vi "pigeon_ver4_1.vi"() -> ()   [LabVIEW 2017]
uses:
  <vilib>/eio/EIONode/EIONode.xnode
  <vilib>/Platform/TimedLoop/XDataNode/XDataNode.xnode
  <vilib>/Platform/TimedLoop/XDataNode/nitl_modes.ctl
  <vilib>/Platform/TimedLoop/XDataNode/XDNodeRunTimeDep.lvlib
  <vilib>/Platform/TimedLoop/XDataNode/wakeup.ctl
  <vilib>/Platform/TimedLoop/XDataNode/timing_clust.ctl
  <vilib>/rvi/DataTransferAndStorage/Container/XNode/niFpgaContainer.xnode
  <vilib>/rvi/eio/common/nirviEmuTemplateMethod_errors.vi
  <vilib>/rvi/Memory/Memory_Emulation/nirvimemoryFastEmulation.vi
  <vilib>/rvi/Memory/Memory_Emulation/nirvimemoryEmulation.vi
  <vilib>/rvi/interface/RandomDataEmulation/nirviRandomDataFpgaReadWriteTemplate.vi
panel:
  out "Numeric":i16
  in  "analog ramp on":bool
  in  "AO5":i16
  out "AI2":i16
  in  "Tab Control":enum32{"pigeon"}(tab)
  out "trigger AI1":bool
  in  "Tab Control 2":T1(tab)
  in  "square wave  on?":bool
  in  "square wave period":i32
  in  "IGBTswitch":bool caption="IGBT Switch circular"
  in  "Manual Override":bool
  in  "circular coil current":i16(slide) scale=0.0..32768.0
  in  "analog ramp period":i16
  in  "AO4":bool
  in  "analog wave shape":i16(ring) items=["Triangle", "Sawtooth", "Sin", ""]
  out "FIFO size":i16
  in  "AO0":i16
  in  "AO1":i16
  in  "AO2":i16
  in  "Run program":bool
  in  "halt processor":bool
  out "control flags":i8 format="%b"
  in  "host operation":i16
  in  "address":u16
  in  "data1":u16
  in  "data2":i32
  in  "repeat program":i32
  out "IP address":i16
  out "PMT1":i16=-4740
  out "ReA":i32
  out "RegB":i16
  out "RegC":i16
  out "exttrigger":bool=TRUE
  out "AI1":i16=161
  out "RegD":i16
  in  "AO4":i16
  in  "AO3":i16
  out "Connector0/AI0":i16
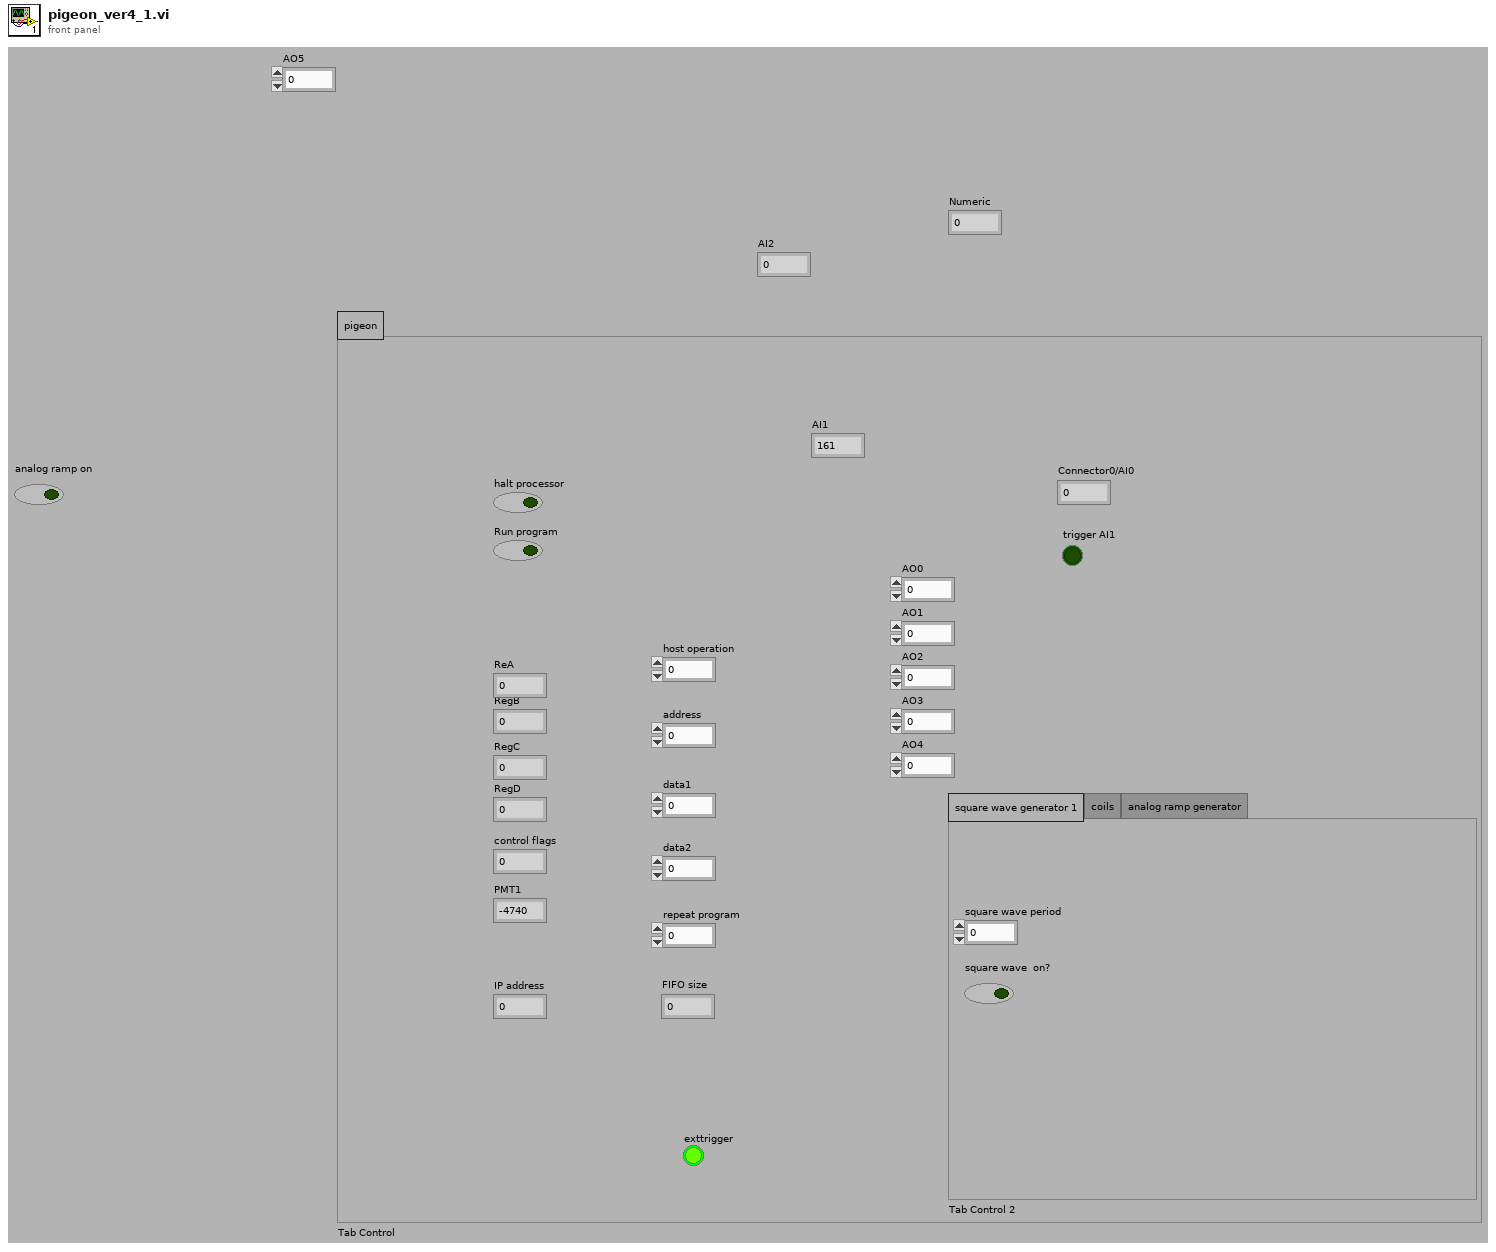
[diagram p1: front panel]
types:
  T1 = enum32{"square wave generator 1", "coils", "analog ramp generator"}
  T2 = typedef "XDNodeRunTimeDep.lvlib/timing_clust.ctl" = cluster{"Expected End [f-1]":u64, "Actual End [f-1]":u64, "Finished Late? [f-1]":bool, "Expected End [i-1]":u64, "Actual End [i-1]":u64, "Finished Late? [i-1]":bool, "Expected Start [i]":u64, "Actual Start [i]":u64, "Expected Start [f]":u64, "Actual Start [f]":u64, "Source Name":string, "Structure Name":string, "Period":i64, "Deadline":i64, "Offset":i64, "Start":i64, "Priority":i32, "Timeout":i32, "Mode":T3, "Wakeup Reason":T4, "Error":errorcluster, "Source Type":string, "Secondary Source Type":string, "Global End Time":u64, "Global Start Time":u64, "Frame Duration":u64, "Iteration Duration":u64, "Assigned CPU":i32, "I/O Scan Engine Mode":u32}
  T3 = typedef "XDNodeRunTimeDep.lvlib/nitl_modes.ctl" = enum32{"No Change", "Process missed periods, maintain original phase", "Discard missed periods, maintain original phase", "Process missed periods, ignore original phase", "Discard missed periods, ignore original phase"}
  T4 = typedef "XDNodeRunTimeDep.lvlib/wakeup.ctl" = enum32{"Normal", "Aborted", "Asynchronous wakeup", "Timing source error", "Timed loop error", "Timeout"}
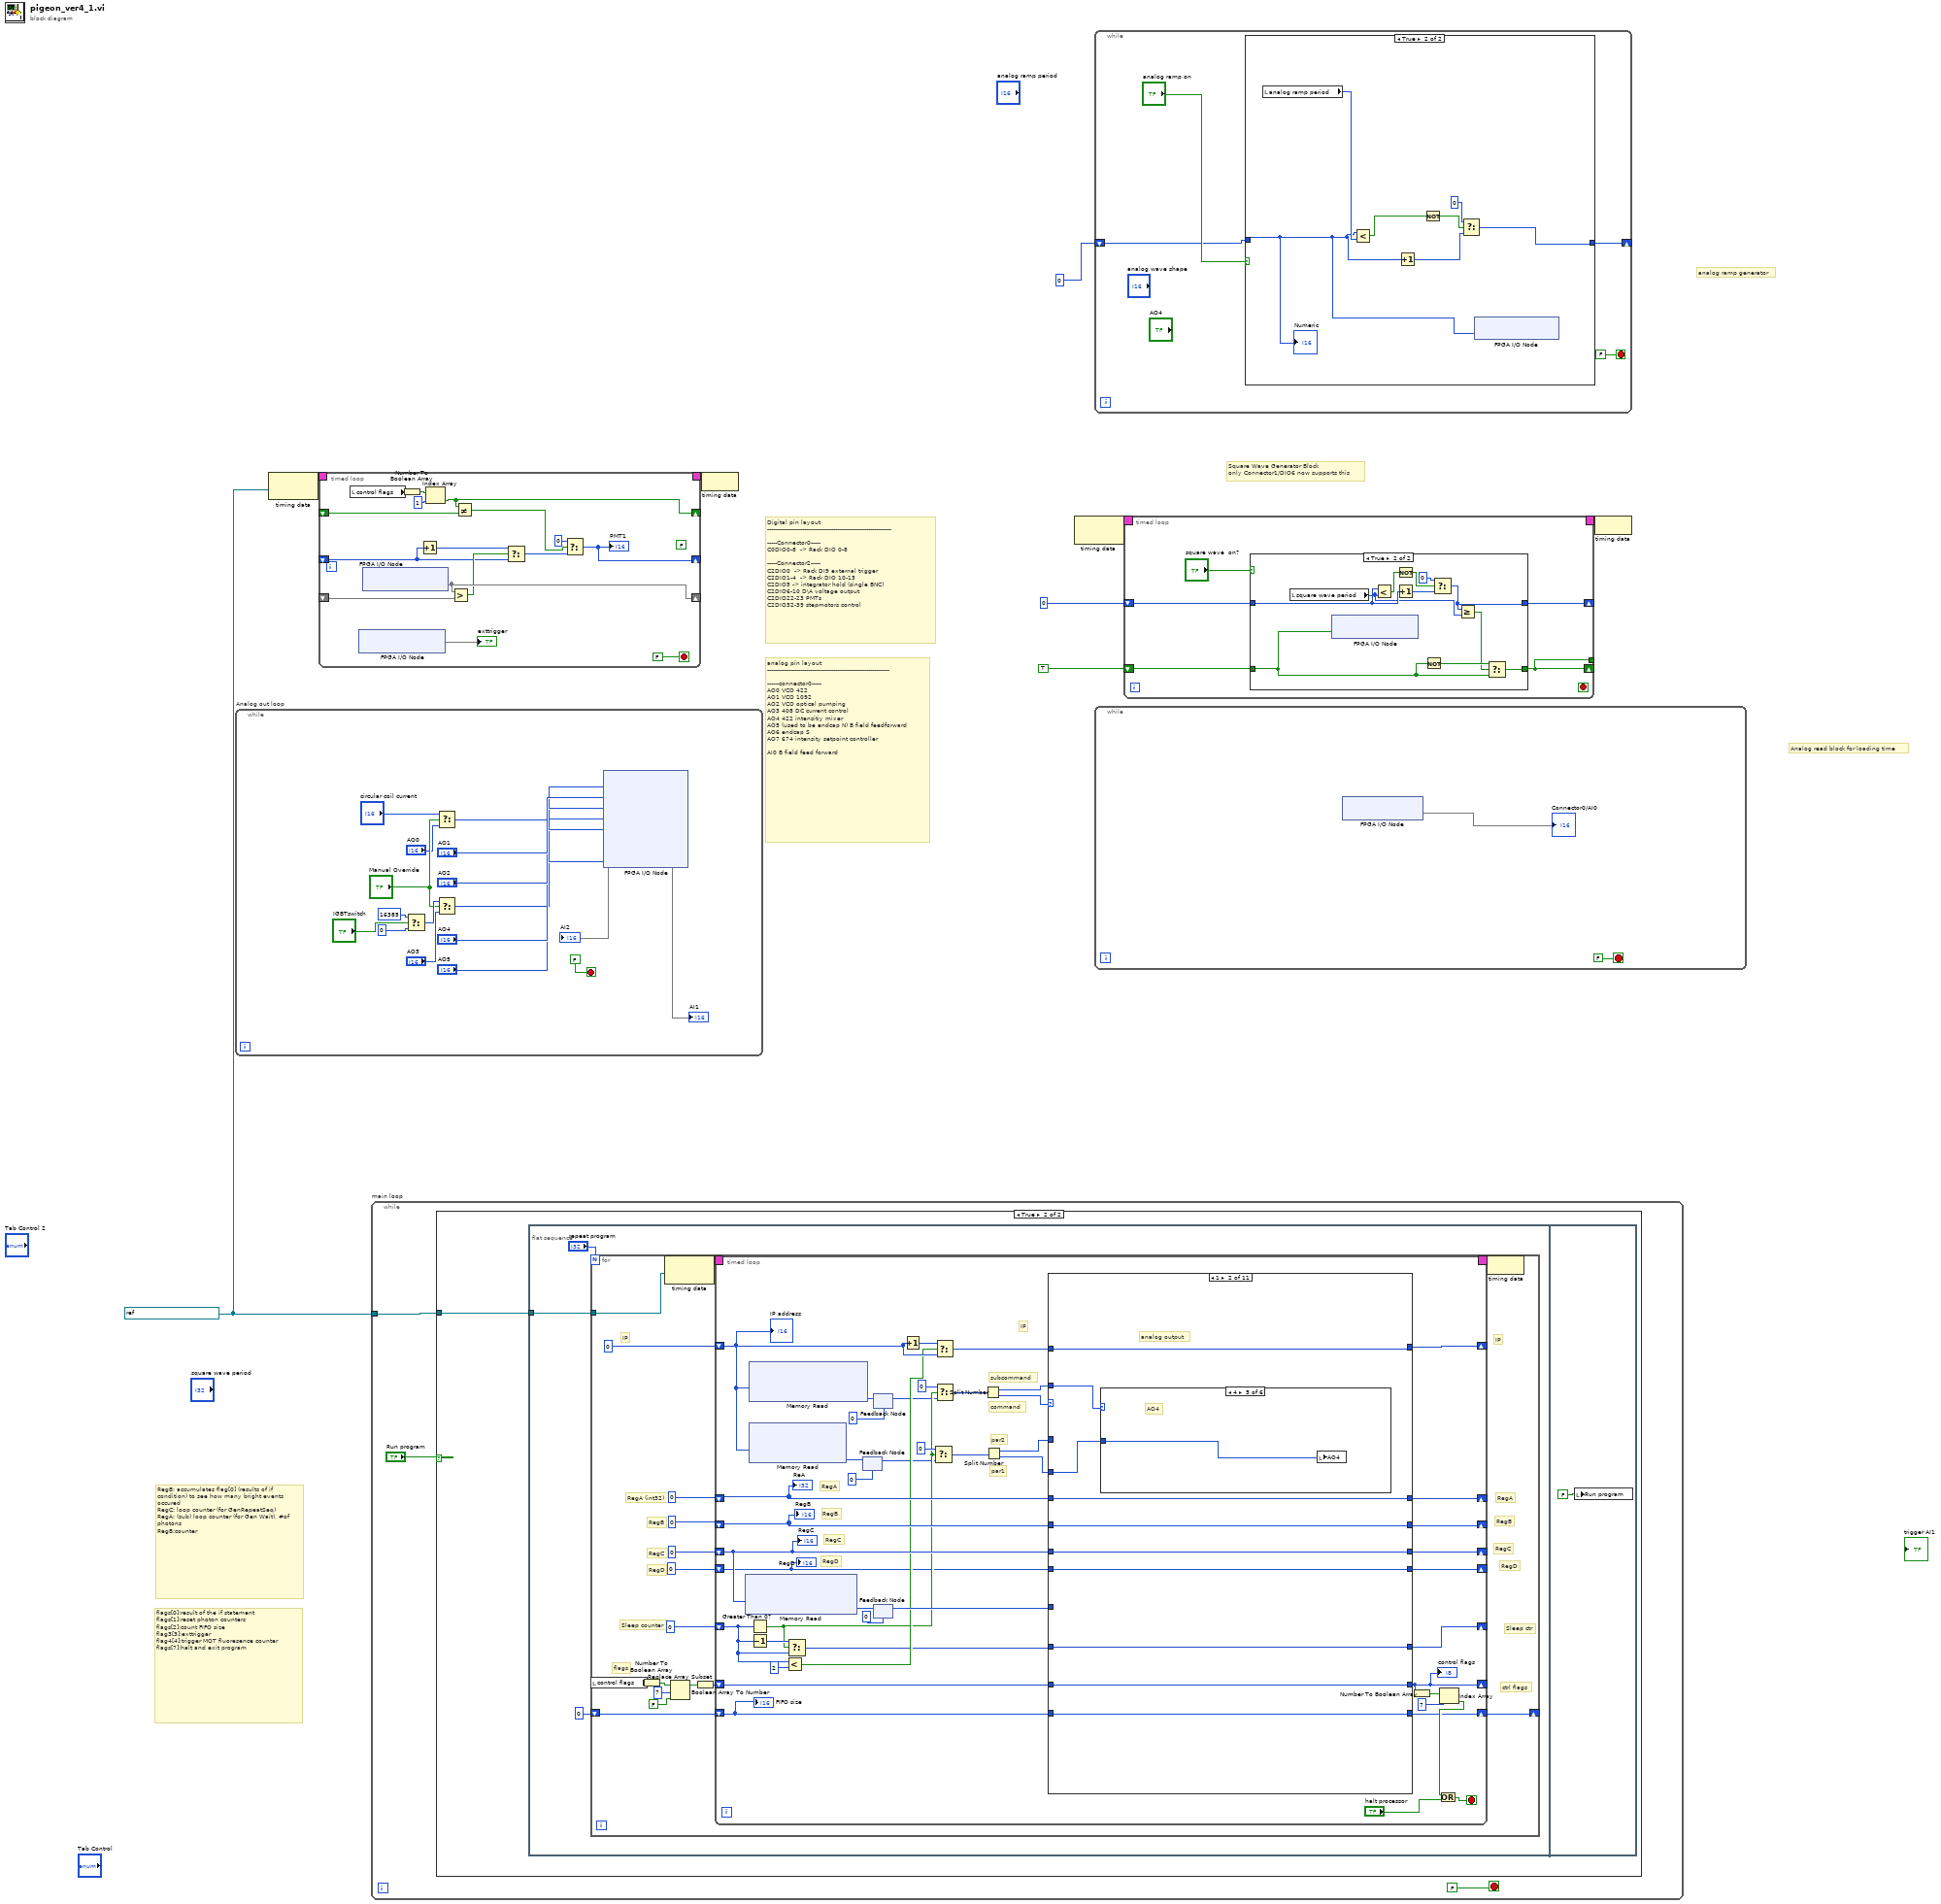
[diagram p0: block diagram]
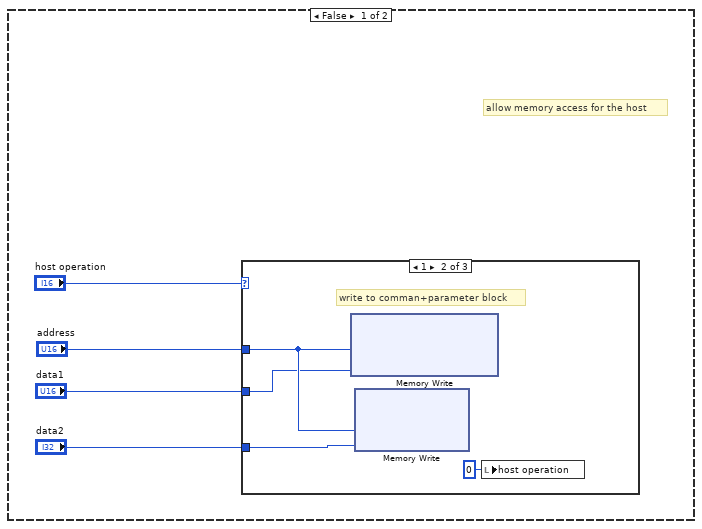
[diagram p4: hidden frame]
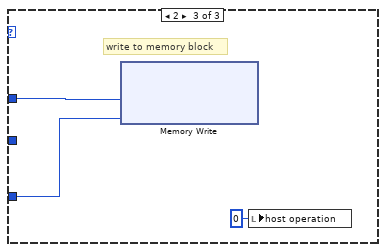
[diagram p6: hidden frame]
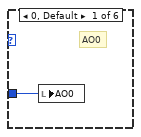
[diagram p8: hidden frame]
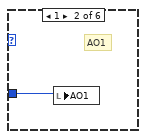
[diagram p9: hidden frame]
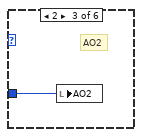
[diagram p10: hidden frame]
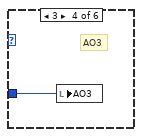
[diagram p11: hidden frame]
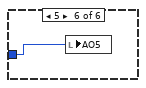
[diagram p12: hidden frame]
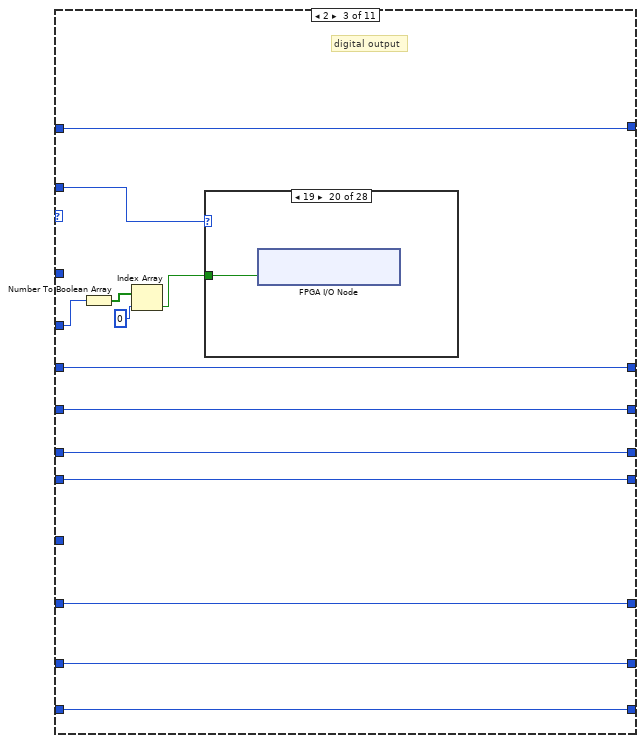
[diagram p13: hidden frame]
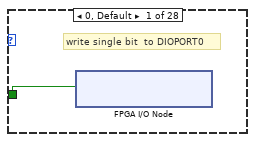
[diagram p14: hidden frame]
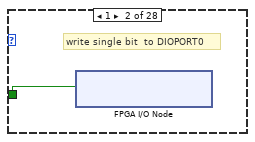
[diagram p15: hidden frame]
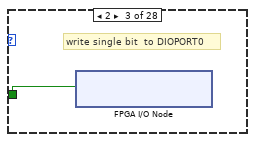
[diagram p16: hidden frame]
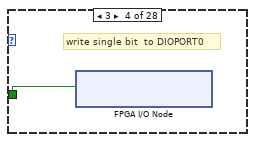
[diagram p17: hidden frame]
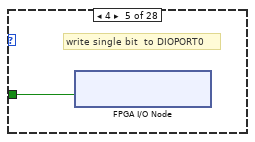
[diagram p18: hidden frame]
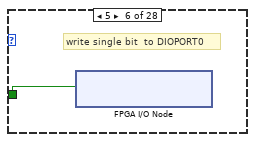
[diagram p19: hidden frame]
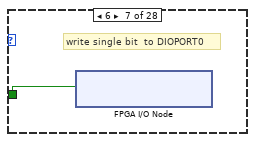
[diagram p20: hidden frame]
diagram:
  w6 = refnum<k21> "40 MHz Onboard Clock" ("FPGA Clock")
  # "analog ramp generator"
  # "Analog read block for loading time"
  # "Square Wave Generator Block\nonly Connector1/DIO6 now supports this"
  # "RegB: accumulates flag[0] (results of if condition) to see how many bright events occured\nRegC: loop counter (for GenRepeatSeq)\nRegA: (sub) loop counter (for Gen Wait), #of     photons \nRegB:counter"
  # "flags[0]:result of the if statement\nflags[1]:reset photon counters\nflags[2]:count FIFO size\nflag3[3]:exttrigger\nflag4[4]:trigger MOT fluoresence counter\nflags[7]:halt and exit program"
  # "Digital pin layout\n----------------------------------------------------------------\n\n-----Connector0-----\nC0DIO0-8  -> Rack DIO 0-8\n\n-----Connector2-----\nC2DIO0  -> Rack DI9 external trigger \nC2DIO1-4  -> Rack DIO 10-13\nC2DIO5 -> integrator hold (single BNC)\nC2DIO6-10 D\\A voltage output\nC2DIO22-23 PMTs\nC2DIO32-39 stepmotors control"
  # "analog pin layout\n---------------------------------------------------------------\n\n------connector0-----\nAO0 VCO 422\nAO1 VCO 1092\nAO2 VCO optical pumping\nAO3 408 DC current control\nAO4 422 intensitiy mixer\nAO5 (used to be endcap N) B field feedforward\nAO6 endcap S\nAO7 674 intensity setpoint controller\n\nAI0 B field feed forward"
  n1 = while "Analog out loop" {
    stop <- FALSE stop-if-true
    n2 = Select(t=i16 16385, s="IGBTswitch", f=i16 0) -> (s? t:f=w15:i16)
    n3 = Select(t="circular coil current", s="Manual Override", f="AO0") -> (s? t:f=w9:i16)
    n4 = Select(t=w15, s="Manual Override", f="AO3") -> (s? t:f=w14:i16)
    n5 = xnode "FPGA I/O Node"("Connector0/AO0"=w9, "Connector0/AO1"="AO1", "Connector0/AO2"="AO2", "Connector0/AO3"=w14, "Connector0/AO4"="AO4", "Connector0/AO5"="AO5") -> ("Connector0/AI1"=→"AI1", "Connector0/AI2"=→"AI2")  [unwired: 8 in, 8 out]
  }
  n6 = node-c288(w6) -> (w8:T2)
  n7 = timed-loop {
    timing: w8 -> [_]
    timing-out: [_] -> w7
    shift-right: [w39] -> _
    shift-left: _ -> [w28]
    shift-right: [w32] -> _
    shift-left: _ -> [w41]
    shift-right: [w34] -> _
    shift-left: _ -> [w35]
    stop <- FALSE stop-if-true
    (unwired) FALSE
    n8 = local read "control flags"() -> (w36:i8)
    n9 = xnode "FPGA I/O Node"() -> ("Connector2/DIO0"=→"exttrigger")  [unwired: 1 in, 1 out]
    n10 = xnode "FPGA I/O Node"() -> ("Connector0/DIO0"=w32)  [unwired: 1 in, 1 out]
    n11 = Number To Boolean Array(number=w36) -> (Boolean array=w37:bool[])
    n12 = Increment(x=w28) -> (x+1=w29:u16)
    n13 = Index Array(array=w37, index=1) -> (element=w34:bool)
    n14 = Greater?(x=w32, y=w41) -> (0:w31:bool)
    n15 = Not Equal?(x=w34, y=w35) -> (x != y?=w26:bool)
    n16 = Select(t=w29, s=w31, f=w28) -> (s? t:f=w40:u16)
    n17 = Select(t=u16 0, s=w26, f=w40) -> (s? t:f=w39:u16)
    "PMT1" <- w39
  }
  n18 = while "main loop" {
    tunnel: w6 -> [w44]
    stop <- FALSE ("stop") stop-if-true
    n19 = case shown="True" "Run program" {
      tunnel: w44 -> [_ w58]
      frame False {
        # "allow memory access for the host"
        n20 = case shown="1" "host operation" {
          tunnel: "address" -> [_ w52 w57]
          tunnel: "data1" -> [_ w51 _]
          tunnel: "data2" -> [_ w54 w55]
          frame 0, Default {
          }
          frame 1 {
            # "write to comman+parameter block"
            n21 = xnode ("Memory Write")("Address"=w52, "Data"=w51) -> ()  [unwired: 1 in, 1 out]
            n22 = xnode ("Memory Write")("Address"=w52, "Data"=w54) -> ()  [unwired: 1 in, 1 out]
            n23 = local write "host operation"(i16 0 ("host operation")) -> ()
          }
          frame 2 {
            # "write to memory block"
            n24 = xnode ("Memory Write")("Address"=w57, "Data"=w55) -> ()  [unwired: 1 in, 1 out]
            n25 = local write "host operation"(i16 0 ("host operation")) -> ()
          }
        }
      }
      frame True {
        n26 = flat-sequence {
          tunnel: w58 -> [w60]
          frame #0 {
            n27 = for {
              N: "repeat program" -> [_]
              tunnel: w60 -> [w72]
              shift-right: [w63] -> _
              shift-left: i16 0 -> [w64]
              # "ctrl flags"
              # "Sleep ctr"
              # "RegD"
              # "RegD"
              # "Sleep counter"
              # "flags"
              # "RegC"
              # "RegB"
              # "RegA"
              # "RegC"
              # "RegB"
              # "RegA (int32)"
              # "IP"
              # "IP"
              n28 = local read "control flags"() -> (w67:i8)
              n29 = Number To Boolean Array(number=w67) -> (Boolean array=w71:bool[])
              n30 = node-c288(w72) -> (w78:T2)
              n31 = Replace Array Subset(array=w71, new element=FALSE ("new element/subarray"), index=7) -> (w69:bool[])
              n32 = Boolean Array To Number(Boolean array=w69) -> (number=w70:u8)
              n33 = timed-loop {
                timing: w78 -> [_]
                timing-out: [_] -> w77
                shift-right: [w113] -> _
                shift-left: i16 0 -> [w96]
                shift-right: [w109] -> _
                shift-left: 0 -> [w105]
                shift-right: [w121] -> _
                shift-left: i16 0 -> [w112]
                shift-right: [w120] -> _
                shift-left: i16 0 -> [w104]
                shift-right: [w110] -> _
                shift-left: w70 -> [w111]
                shift-right: [w103] -> _
                shift-left: i16 0 -> [w94]
                shift-right: [w85] -> w63
                shift-left: w64 -> [w84]
                shift-right: [w82] -> _
                shift-left: i16 0 -> [w83]
                stop <- w116 stop-if-true
                # "RegD"
                # "IP"
                # "RegC"
                # "RegB"
                # "RegA"
                # "par1"
                # "par2"
                # "subcommand"
                # "command"
                n34 = xnode ("Memory Read")("Address"=w104) -> ("Data"=w108:i16)  [unwired: 2 in, 2 out]
                n35 = xnode ("Memory Read")("Address"=w96) -> ("Data"=w91:u16)  [unwired: 1 in, 1 out]
                n36 = xnode ("Memory Read")("Address"=w96) -> ("Data"=w87:i32)  [unwired: 1 in, 1 out]
                n37 = Greater Than 0?(x=w94) -> (x > 0?=w89:bool)
                n38 = Decrement(x=w94) -> (x-1=w95:u32)
                n39 = Less?(x=w94, y=u32 2) -> (x < y?=w93:bool)
                n40 = Select(t=w95, s=w89, f=w94) -> (s? t:f=w92:u32)
                n41 = feedback-in #1(w87) -> ()
                n42 = feedback #1(u32 0 ("Data")) -> (w86:u32)
                n43 = feedback-in #2(w108) -> ()
                n44 = feedback #2(0) -> (w107:i32)
                n45 = feedback-in #3(w91) -> ()
                n46 = feedback #3(u16 0 ("Data")) -> (w88:u16)
                n47 = Increment(x=w96) -> (x+1=w97:u16)
                n48 = Select(t=0, s=w89, f=w86) -> (s? t:f=w100:u32)
                n49 = Select(t=w97, s=w93, f=w96) -> (s? t:f=w102:u16)
                n50 = Select(t=u16 0, s=w89, f=w88) -> (s? t:f=w101:u16)
                n51 = Split Number(x=w101) -> (hi(x)=w122:u8, lo(x)=w123:u8)
                n52 = Split Number(x=w100) -> (hi(x)=w114:u16, lo(x)=w115:u16)
                n53 = case shown="1" w123 {
                  tunnel: w115 -> [_ w140 w152 _ w232 w352 w426 _ _ w485 _]
                  tunnel: w114 -> [_ _ _ _ w225 w351 w425 _ _ w486 _]
                  tunnel: w122 -> [_ w141 w160 w199 w233 w356 _ w444 _ w468 _]
                  tunnel: w105 -> [w131 w139 w159 w191 w231 w353 w430 w448 w464 w484 w503]
                  tunnel: [w131 w139 w159 w191 w228 w353 w430 w448 w464 w483 w503] -> w109
                  tunnel: w112 -> [w130 w138 w158 w190 w230 w354 w431 w447 w467 w482 w504]
                  tunnel: w104 -> [w129 w137 w157 w197 w229 w355 w432 w446 w466 w480 w505]
                  tunnel: [w130 w138 w158 w189 w227 w354 w431 w447 w467 w481 w504] -> w121
                  tunnel: [w129 w137 w157 w197 w226 w355 w432 w446 w466 w479 w505] -> w120
                  tunnel: [w127 w136 w156 w198 w221 w359 w424 w450 w465 w469 w502] -> w113
                  tunnel: w102 -> [w127 w136 w156 w198 w222 w359 _ w450 w465 w470 w502]
                  tunnel: [w128 w135 w155 w195 w223 w358 w423 w439 w461 w473 w508] -> w110
                  tunnel: w111 -> [w128 w135 w155 w196 w224 w357 w423 w438 w460 w474 w508]
                  tunnel: w107 -> [_ _ _ _ w215 w350 _ _ _ _ _]
                  tunnel: w92 -> [w126 w134 w150 w194 w220 w349 w422 w436 w457 w476 w509]
                  tunnel: [w126 w134 w150 w194 w219 w349 w422 w436 w457 w475 w509] -> w103
                  tunnel: w84 -> [w125 w133 w149 w193 w218 w348 w421 w435 w456 w471 w507]
                  tunnel: [w125 w133 w149 w193 w218 w348 w421 w434 w456 w472 w507] -> w85
                  tunnel: w83 -> [w124 w132 w148 w192 w217 w347 w420 w433 w455 w478 w506]
                  tunnel: [w124 w132 w148 w192 w216 w347 w420 w433 w455 w477 w506] -> w82
                  frame 0, Default {
                  }
                  frame 1 {
                    # "analog output"
                    n54 = case shown="4" w141 {
                      tunnel: w140 -> [w142 w143 w144 w145 w146 w147]
                      frame 0, Default {
                        # "AO0"
                        n55 = local write "AO0"(w142) -> ()
                      }
                      frame 1 {
                        # "AO1"
                        n56 = local write "AO1"(w143) -> ()
                      }
                      frame 2 {
                        # "AO2"
                        n57 = local write "AO2"(w144) -> ()
                      }
                      frame 3 {
                        # "AO3"
                        n58 = local write "AO3"(w145) -> ()
                      }
                      frame 4 {
                        # "AO4"
                        n59 = local write "AO4"(w146) -> ()
                      }
                      frame 5 {
                        n60 = local write "AO5"(w147) -> ()
                      }
                    }
                  }
                  frame 2 {
                    # "digital output"
                    n61 = Number To Boolean Array(number=w152) -> (Boolean array=w153:bool[])
                    n62 = Index Array(array=w153, index=0) -> (element=w151:bool)
                    n63 = case shown="19" w160 {
                      tunnel: w151 -> [w161 w162 w163 w164 w165 w166 w167 w168 w169 w170 w171 w172 w173 w174 w175 w176 w177 w178 w179 w180 w181 w182 w183 w184 w185 w186 w187 w188]
                      frame 0, Default {
                        # "write single bit  to DIOPORT0"
                        n64 = xnode "FPGA I/O Node"("Connector1/DIO0"=w161) -> ()  [unwired: 1 in, 1 out]
                      }
                      frame 1 {
                        # "write single bit  to DIOPORT0"
                        n65 = xnode "FPGA I/O Node"("Connector1/DIO1"=w162) -> ()  [unwired: 1 in, 1 out]
                      }
                      frame 2 {
                        # "write single bit  to DIOPORT0"
                        n66 = xnode "FPGA I/O Node"("Connector1/DIO2"=w163) -> ()  [unwired: 1 in, 1 out]
                      }
                      frame 3 {
                        # "write single bit  to DIOPORT0"
                        n67 = xnode "FPGA I/O Node"("Connector1/DIO3"=w164) -> ()  [unwired: 1 in, 1 out]
                      }
                      frame 4 {
                        # "write single bit  to DIOPORT0"
                        n68 = xnode "FPGA I/O Node"("Connector1/DIO4"=w165) -> ()  [unwired: 1 in, 1 out]
                      }
                      frame 5 {
                        # "write single bit  to DIOPORT0"
                        n69 = xnode "FPGA I/O Node"("Connector1/DIO5"=w166) -> ()  [unwired: 1 in, 1 out]
                      }
                      frame 6 {
                        # "write single bit  to DIOPORT0"
                        n70 = xnode "FPGA I/O Node"("Connector1/DIO6"=w167) -> ()  [unwired: 1 in, 1 out]
                      }
                      frame 7 {
                        # "write single bit  to DIOPORT0"
                        n71 = xnode "FPGA I/O Node"("Connector1/DIO7"=w168) -> ()  [unwired: 1 in, 1 out]
                      }
                      frame 8 {
                        # "write single bit  to DIOPORT0"
                        n72 = xnode "FPGA I/O Node"("Connector1/DIO8"=w169) -> ()  [unwired: 1 in, 1 out]
                      }
                      frame 9 {
                        n73 = xnode "FPGA I/O Node"("Connector1/DIO9"=w170) -> ()  [unwired: 1 in, 1 out]
                      }
                      frame 10 {
                        n74 = xnode "FPGA I/O Node"("Connector1/DIO10"=w171) -> ()  [unwired: 1 in, 1 out]
                      }
                      frame 11 {
                        n75 = xnode "FPGA I/O Node"("Connector1/DIO11"=w172) -> ()  [unwired: 1 in, 1 out]
                      }
                      frame 12 {
                        n76 = xnode "FPGA I/O Node"("Connector1/DIO12"=w173) -> ()  [unwired: 1 in, 1 out]
                      }
                      frame 13 {
                        n77 = xnode "FPGA I/O Node"("Connector1/DIO13"=w174) -> ()  [unwired: 1 in, 1 out]
                      }
                      frame 14 {
                        n78 = xnode "FPGA I/O Node"("Connector1/DIO14"=w175) -> ()  [unwired: 1 in, 1 out]
                      }
                      frame 15 {
                        n79 = xnode "FPGA I/O Node"("Connector1/DIO15"=w176) -> ()  [unwired: 1 in, 1 out]
                      }
                      frame 16 {
                        n80 = xnode "FPGA I/O Node"("Connector1/DIO16"=w177) -> ()  [unwired: 1 in, 1 out]
                      }
                      frame 17 {
                        n81 = xnode "FPGA I/O Node"("Connector1/DIO17"=w178) -> ()  [unwired: 1 in, 1 out]
                      }
                      frame 18 {
                        n82 = xnode "FPGA I/O Node"("Connector1/DIO18"=w179) -> ()  [unwired: 1 in, 1 out]
                      }
                      frame 19 {
                        n83 = xnode "FPGA I/O Node"("Connector1/DIO19"=w180) -> ()  [unwired: 1 in, 1 out]
                      }
                      frame 20 {
                        n84 = xnode "FPGA I/O Node"("Connector2/DIO12"=w181) -> ()  [unwired: 1 in, 1 out]
                      }
                      frame 21 {
                        n85 = xnode "FPGA I/O Node"("Connector2/DIO17"=w182) -> ()  [unwired: 1 in, 1 out]
                      }
                      frame 22 {
                        n86 = xnode "FPGA I/O Node"("Connector2/DIO19"=w183) -> ()  [unwired: 1 in, 1 out]
                      }
                      frame 23 {
                        n87 = xnode "FPGA I/O Node"("Connector2/DIO18"=w184) -> ()  [unwired: 1 in, 1 out]
                      }
                      frame 24 {
                        n88 = xnode "FPGA I/O Node"("Connector2/DIO21"=w185) -> ()  [unwired: 1 in, 1 out]
                      }
                      frame 25 {
                        n89 = xnode "FPGA I/O Node"("Connector2/DIO24"=w186) -> ()  [unwired: 1 in, 1 out]
                      }
                      frame 26 {
                        n90 = xnode "FPGA I/O Node"("Connector2/DIO25"=w187) -> ()  [unwired: 1 in, 1 out]
                      }
                      frame 27 {
                        n91 = xnode "FPGA I/O Node"("Connector2/DIO20"=w188) -> ()  [unwired: 1 in, 1 out]
                      }
                    }
                  }
                  frame 3 {
                    # "photon counting"
                    n92 = case shown="3" w199 {
                      tunnel: [w200 w202 w214] -> w189
                      tunnel: w190 -> [w200 w203 w214]
                      tunnel: w196 -> [w201 w205 w212]
                      tunnel: [w201 w205 w211] -> w195
                      frame 2, Default {
                      }
                      frame 1 {
                        # "PMT1"
                        n93 = local read "PMT1"() -> (w204:i16)
                        n94 = Add(x=w204, y=w203) -> (x+y=w202:u16)
                      }
                      frame 3 {
                        # "Reset  photon counter"
                        # "make a Not gate of flag(1)"
                        n95 = Number To Boolean Array(number=w212) -> (Boolean array=w209:bool[])
                        n96 = Index Array(array=w209, index=1) -> (element=w207:bool)
                        n97 = Not(x=w207) -> (.not. x?=w206:bool)
                        n98 = Replace Array Subset(array=w209, new element=w206, index=1) -> (w210:bool[])
                        n99 = Boolean Array To Number(Boolean array=w210) -> (number=w211:u8)
                      }
                    }
                  }
                  frame 4 {
                    # "registers operation"
                    n100 = case shown="7" w233 {
                      tunnel: w232 -> [w239 w249 w256 _ _ _ _ w298 _ _ w325 w338]
                      tunnel: w231 -> [_ w248 w255 w262 w270 w278 w282 w303 w314 w320 w330 w343]
                      tunnel: w230 -> [w242 _ w254 w261 w272 w277 w290 w302 w313 w316 w328 w341]
                      tunnel: w229 -> [w241 w247 _ w264 w271 _ w283 w301 w312 w319 w329 w342]
                      tunnel: [w238 w248 w255 w262 w269 w278 w282 w303 w314 w320 w330 w343] -> w228
                      tunnel: [w242 w249 w254 w261 w272 w277 w289 w302 w313 w318 w328 w341] -> w227
                      tunnel: [w241 w247 w256 w263 w271 w277 w283 w301 w312 w319 w329 w342] -> w226
                      tunnel: w225 -> [w240 _ _ _ _ _ _ w299 _ _ _ w337]
                      tunnel: w224 -> [w237 w246 w253 w260 w268 w276 w284 w300 w311 w323 w333 w346]
                      tunnel: [w237 w246 w253 w260 w268 w276 w284 w300 w311 w323 w333 w346] -> w223
                      tunnel: w222 -> [w236 w245 w252 w259 w267 w275 w281 w292 w306 w322 w332 w345]
                      tunnel: [w236 w245 w252 w259 w267 w275 w281 w295 w309 w322 w332 w345] -> w221
                      tunnel: w220 -> [w235 w244 w251 w258 w266 w274 w280 _ _ w321 w331 w344]
                      tunnel: [w235 w244 w251 w258 w266 w274 w280 w296 w304 w321 w331 w344] -> w219
                      tunnel: w217 -> [w234 w243 w250 w257 w265 w273 w279 w291 w305 w315 _ w336]
                      tunnel: [w234 w243 w250 w257 w265 w273 w279 w291 w305 w315 w326 w335] -> w216
                      tunnel: w215 -> [_ _ _ _ _ _ _ _ w304 _ _ _]
                      frame 0, Default {
                        # "Set par1,2 to RegA"
                        n101 = Join Numbers(hi=w240, lo=w239) -> ((hi.lo)=w238:u32)
                      }
                      frame 1 {
                        # "Set par1 to RegB"
                      }
                      frame 2 {
                        # "Set par1 to RegC"
                      }
                      frame 3 {
                        # "increase RegC by 1"
                        n102 = Increment(x=w264) -> (x+1=w263:u16)
                      }
                      frame 4 {
                        # "increase RegA by 1"
                        n103 = Increment(x=w270) -> (x+1=w269:u32)
                      }
                      frame 5 {
                        # "Set regC to regB"
                      }
                      frame 6 {
                        # "regB<-regB+flags[0]"
                        n104 = Number To Boolean Array(number=w284) -> (Boolean array=w288:bool[])
                        n105 = Index Array(array=w288, index=0) -> (element=w286:bool)
                        n106 = Boolean To (0,1)(Boolean=w286) -> (0, 1=w285:i16)
                        n107 = Add(x=w285, y=w290) -> (x+y=w289:u16)
                      }
                      frame 7 {
                        # "Sleep counter = [par1 par2]"
                        n108 = Join Numbers(hi=w299, lo=w298) -> ((hi.lo)=w296:u32)
                        n109 = Greater?(x=w296, y=u32 0) -> (0:w294:bool)
                        n110 = Decrement(x=w292) -> (x-1=w293:u16)
                        n111 = Select(t=w293, s=w294, f=w292) -> (s? t:f=w295:u16)
                      }
                      frame 11 {
                        # "Sleep counter =par1* memory Block[RegC]"
                        n112 = Greater?(x=w304, y=u32 0) -> (0:w308:bool)
                        n113 = Decrement(x=w306) -> (x-1=w307:u16)
                        n114 = Select(t=w307, s=w308, f=w306) -> (s? t:f=w309:u16)
                      }
                      frame 8 {
                        # "RegB=RegB+ RegA(lo)"
                        n115 = Split Number(x=w320) -> (lo(x)=w317:u16)  [unwired: 1 out]
                        n116 = Add(x=w317, y=w316) -> (x+y=w318:u16)
                      }
                      frame 9 {
                        # "RegD<-AI1+par1"
                        n117 = To Word Integer(number=w325) -> (16bit integer=w324:i16)
                        n118 = local read "AI1"() -> (w327:i16)
                        n119 = Add(x=w324, y=w327) -> (x+y=w326:i16)
                      }
                      frame 10 {
                        # "RegD<-RegD*2^par1*par2"
                        n120 = To Word Integer(number=w337) -> (16bit integer=w339:i16)
                        n121 = To Word Integer(number=w338) -> (16bit integer=w340:i16)
                        n122 = Multiply(x=w339, y=w336) -> (x*y=w334:i16)
                        n123 = Scale By Power Of 2(n=w340, x=w334) -> (x*2^n=w335:i16)
                      }
                    }
                  }
                  frame 5 {
                    # "If statement"
                    n124 = case shown="4" w356 {
                      tunnel: [w369 w377 w385 w393 w403 w406 w414] -> w358
                      tunnel: w357 -> [w368 w376 w384 w392 w402 w407 w415]
                      tunnel: w351 -> [w362 _ _ _ _ _ _]
                      tunnel: w355 -> [_ _ w380 w387 _ _ _]
                      tunnel: w354 -> [_ w371 _ w386 _ _ _]
                      tunnel: w353 -> [w363 _ _ _ _ w404 w412]
                      tunnel: w352 -> [w361 w370 w379 _ _ w405 _]
                      tunnel: w350 -> [_ _ _ _ _ _ w419]
                      frame 0, Default {
                        # "The if regA =  [par1,par2]"
                        n125 = Number To Boolean Array(number=w368) -> (Boolean array=w366:bool[])
                        n126 = Join Numbers(hi=w362, lo=w361) -> ((hi.lo)=w360:u32)
                        n127 = Equal?(x=w360, y=w363) -> (x = y?=w364:bool)
                        n128 = Replace Array Subset(array=w366, new element=w364, index=0) -> (w365:bool[])
                        n129 = Boolean Array To Number(Boolean array=w365) -> (number=w369:u8)
                      }
                      frame 1 {
                        # "The if  regB >  par1"
                        n130 = Number To Boolean Array(number=w376) -> (Boolean array=w374:bool[])
                        n131 = Greater?(x=w371, y=w370) -> (0:w372:bool)
                        n132 = Replace Array Subset(array=w374, new element=w372, index=0) -> (w373:bool[])
                        n133 = Boolean Array To Number(Boolean array=w373) -> (number=w377:u8)
                      }
                      frame 2 {
                        # "The if  regC=  par1"
                        n134 = Number To Boolean Array(number=w384) -> (Boolean array=w382:bool[])
                        n135 = Equal?(x=w379, y=w380) -> (x = y?=w378:bool)
                        n136 = Replace Array Subset(array=w382, new element=w378, index=0) -> (w381:bool[])
                        n137 = Boolean Array To Number(Boolean array=w381) -> (number=w385:u8)
                      }
                      frame 3 {
                        # "The if  regB> regC"
                        n138 = Number To Boolean Array(number=w392) -> (Boolean array=w390:bool[])
                        n139 = Greater?(x=w386, y=w387) -> (0:w388:bool)
                        n140 = Replace Array Subset(array=w390, new element=w388, index=0) -> (w389:bool[])
                        n141 = Boolean Array To Number(Boolean array=w389) -> (number=w393:u8)
                      }
                      frame 4 {
                        w398 = 3 ("index")
                        # "external trigger rising edge"
                        n142 = Number To Boolean Array(number=w402) -> (Boolean array=w399:bool[])
                        n143 = local read "exttrigger"() -> (w395:bool)
                        n144 = Index Array(array=w399, index=w398) -> (element=w397:bool)
                        n145 = Not(x=w397) -> (.not. x?=w396:bool)
                        n146 = And(x=w395, y=w396) -> (x .and. y?=w394:bool)
                        n147 = Replace Array Subset(array=w399, new element #1=w394, index #1=0 ("index"), new element #2=w395, index #2=w398) -> (w400:bool[])
                        n148 = Boolean Array To Number(Boolean array=w400) -> (number=w403:u8)
                      }
                      frame 5 {
                        # "The if  regA >  par1"
                        n149 = Number To Boolean Array(number=w407) -> (Boolean array=w410:bool[])
                        n150 = Greater?(x=w404, y=w405) -> (0:w408:bool)
                        n151 = Replace Array Subset(array=w410, new element=w408, index=0) -> (w409:bool[])
                        n152 = Boolean Array To Number(Boolean array=w409) -> (number=w406:u8)
                      }
                      frame 6 {
                        # "The if  regA == memoryBlock(regC)"
                        n153 = Number To Boolean Array(number=w415) -> (Boolean array=w417:bool[])
                        n154 = Equal?(x=w412, y=w419) -> (x = y?=w413:bool)
                        n155 = Replace Array Subset(array=w417, new element=w413, index=0) -> (w416:bool[])
                        n156 = Boolean Array To Number(Boolean array=w416) -> (number=w414:u8)
                      }
                    }
                  }
                  frame 6 {
                    # "condition (flags[0]) goto\nuse par1=par2 for normal goto"
                    n157 = Number To Boolean Array(number=w423) -> (Boolean array=w429:bool[])
                    n158 = Index Array(array=w429, index=0) -> (element=w427:bool)
                    n159 = Select(t=w426, s=w427, f=w425) -> (s? t:f=w424:u16)
                  }
                  frame 7 {
                    w437 = 2 ("index")
                    # "make a Not gate of flag(2)"
                    # "push  to FIFO"
                    n160 = case shown="4" w444 {
                      tunnel: w448 -> [w451 _ _ _]
                      tunnel: w447 -> [_ w452 _ _]
                      tunnel: w446 -> [_ _ w453 _]
                      tunnel: [w451 w452 w453 w454] -> w445
                      frame 0, Default {
                        # "push RegA"
                      }
                      frame 1 {
                        # "push RegB"
                      }
                      frame 2 {
                        # "push RegC"
                      }
                      frame 4 {
                        n161 = local read "AI1"() -> (w454:i16)
                      }
                    }
                    n162 = Number To Boolean Array(number=w438) -> (Boolean array=w442:bool[])
                    n163 = Index Array(array=w442, index=w437) -> (element=w441:bool)
                    n164 = Not(x=w441) -> (.not. x?=w440:bool)
                    n165 = Replace Array Subset(array=w442, new element=w440, index=w437) -> (w443:bool[])
                    n166 = Increment(x=w435) -> (x+1=w434:i16)
                    n167 = Boolean Array To Number(Boolean array=w443) -> (number=w439:u8)
                    n168 = xnode ("FIFO Write")("Element"=w445, "Timeout"=0) -> ()  [unwired: 1 in, 2 out]
                  }
                  frame 8 {
                    # "Stop and reset program"
                    n169 = Number To Boolean Array(number=w460) -> (Boolean array=w463:bool[])
                    n170 = Replace Array Subset(array=w463, new element=TRUE ("new element/subarray"), index=7) -> (w462:bool[])
                    n171 = Boolean Array To Number(Boolean array=w462) -> (number=w461:u8)
                  }
                  frame 9 {
                    # "Cold Lab Specific instructions"
                    n172 = case shown="0, Default" w468 {
                      tunnel: w486 -> [w499]
                      tunnel: w485 -> [w498]
                      tunnel: w468 -> [w497]
                      tunnel: w484 -> [w494]
                      tunnel: [w494] -> w483
                      tunnel: w482 -> [w493]
                      tunnel: [w493] -> w481
                      tunnel: w480 -> [w492]
                      tunnel: [w492] -> w479
                      tunnel: w478 -> [w491]
                      tunnel: [w491] -> w477
                      tunnel: w476 -> [w490]
                      tunnel: [w490] -> w475
                      tunnel: w474 -> [w489]
                      tunnel: [w489] -> w473
                      tunnel: [w488] -> w472
                      tunnel: w471 -> [w488]
                      tunnel: w470 -> [w487]
                      tunnel: [w487] -> w469
                      frame 0, Default {
                        # "Run Square wave generator"
                        n173 = Greater?(x=w497, y=u8 0) -> (0:w495:bool)
                        n174 = Join Numbers(hi=w499, lo=w498) -> ((hi.lo)=w500:u32)
                        n175 = local write "square wave  on?"(w495) -> ()
                        n176 = local write "square wave period"(w500) -> ()
                      }
                    }
                  }
                  frame 10 {
                    n177 = local write "trigger AI1"(TRUE) -> ()
                  }
                }
                "control flags" <- w110
                n178 = Number To Boolean Array(number=w110) -> (Boolean array=w119:bool[])
                n179 = Index Array(array=w119, index=7) -> (element=w117:bool)
                n180 = Or(x=w117, y="halt processor") -> (x .or. y?=w116:bool)
                "IP address" <- w96
                "ReA" <- w105
                "RegB" <- w112
                "RegC" <- w104
                "FIFO size" <- w84
                "RegD" <- w83
              }
              n181 = node-c288(w77) -> ()
            }
          }
          frame #1 {
            n182 = local write "Run program"(FALSE ("Run program")) -> ()
          }
        }
      }
    }
  }
  n183 = node-c288(w7) -> ()
  n184 = node-c288() -> (w5:T2)  [unwired: 1 in]
  n185 = while {
    shift-right: [w517] -> _
    shift-left: i16 0 -> [w518]
    stop <- FALSE stop-if-true
    n186 = case shown="True" "analog ramp on" {
      tunnel: [w521 w525] -> w517
      tunnel: w518 -> [w521 w522]
      frame False {
      }
      frame True {
        n187 = local read "analog ramp period"() -> (w524:i16)
        n188 = Less?(x=w522, y=w524) -> (x < y?=w523:bool)
        n189 = Increment(x=w522) -> (x+1=w526:i16)
        n190 = Not(x=w523) -> (.not. x?=w528:bool)
        n191 = Select(t=i16 0, s=w528, f=w526) -> (s? t:f=w525:i16)
        n192 = xnode "FPGA I/O Node"("Connector0/AO7"=w522) -> ()  [unwired: 1 in, 1 out]
        "Numeric" <- w522
      }
    }
  }
  n193 = while {
    stop <- FALSE stop-if-true
    n194 = xnode "FPGA I/O Node"() -> ("Connector0/AI0"=→"Connector0/AI0")  [unwired: 1 in, 1 out]
  }
  n195 = timed-loop {
    shift-right: [w532] -> _
    shift-left: u64 0 -> [w535]
    shift-right: [w534] -> _
    shift-left: TRUE -> [w533]
    timing: w5 -> [_]
    timing-out: [_] -> w4
    tunnel: [w534] -> _
    stop <- _ stop-if-true
    n196 = case shown="True" "square wave  on?" {
      tunnel: w535 -> [w537 w541]
      tunnel: [w536 w545] -> w534
      tunnel: w533 -> [w536 w544]
      tunnel: [w537 w542] -> w532
      frame False {
      }
      frame True {
        n197 = local read "square wave period"() -> (w540:i32)
        n198 = xnode "FPGA I/O Node"("Connector1/DIO6"=w544) -> ()  [unwired: 1 in, 1 out]
        n199 = Less?(x=w541, y=w540) -> (x < y?=w538:bool)
        n200 = Not(x=w538) -> (.not. x?=w539:bool)
        n201 = Increment(x=w541) -> (x+1=w547:u64)
        n202 = Not(x=w544) -> (.not. x?=w546:bool)
        n203 = Select(t=i16 0, s=w539, f=w547) -> (s? t:f=w542:u64)
        n204 = Greater Or Equal?(x=w542, y=w540) -> (x >= y?=w543:bool)
        n205 = Select(t=w546, s=w543, f=w544) -> (s? t:f=w545:bool)
      }
    }
  }
  n206 = node-c288(w4) -> ()
